vi "writeU16.vi"(8 "error in (no error)":errorcluster, 10 "Input":u16, 11 "ModbusBuffer in":refnum<class "ModbusBuffer.lvclass">) -> (0 "error out":errorcluster, 3 "ModbusBuffer out":refnum<class "ModbusBuffer.lvclass">)   [LabVIEW 2016, in "RTModbus.lvlib" / "ModbusBuffer.lvclass"]
uses:
  ModbusBuffer.lvclass
  ModbusBuffer.lvclass/ModbusBuffer.ctl
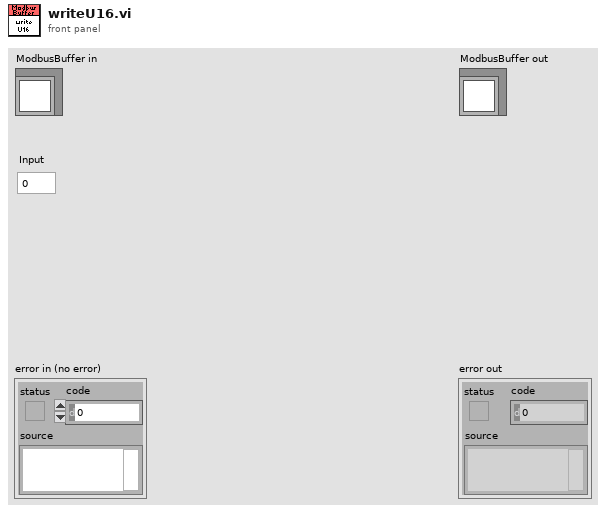
[diagram p1: front panel]
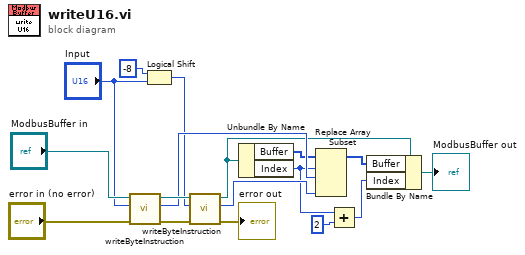
[diagram p0: block diagram]
diagram:
  n1 = call "writeByteInstruction.vi"("error in (no error)"="error in (no error)", "Input"="Input", "ModbusBuffer in"="ModbusBuffer in") -> ("error out"=w6:errorcluster, "Output"=w10:u16, "ModbusBuffer out"=w12:refnum<class "ModbusBuffer.lvclass">)  [unwired: 6 in]
  n2 = Logical Shift(y=i16 -8, x="Input") -> (x << y=w8:u16)
  n3 = call "writeByteInstruction.vi"("error in (no error)"=w6, "Input"=w8, "ModbusBuffer in"=w12) -> ("error out"=→"error out":errorcluster, "Output"=w9:u16, "ModbusBuffer out"=w5:refnum<class "ModbusBuffer.lvclass">)  [unwired: 6 in]
  n4 = Unbundle By Name(w5) -> ("Buffer"=w3:u16[], "Index"=w2:i32)
  n5 = Replace Array Subset(array=w3, new element #1=w10, index #1=w2, new element #2=w9) -> (w14:u16[])  [unwired: 1 in]
  n6 = Add(x=w2, y=2) -> (x+y=w16:i32)
  n7 = Bundle By Name(cluster=w5, "Buffer"=w14, "Index"=w16) -> (→"ModbusBuffer out":refnum<class "ModbusBuffer.lvclass">)
